vi "CRYChange Post Processing Data.vi"(8 "Step Setup VI No":i32, 9 "New Name":string[](array[string]), 10 "Old Name":string[](array[string]), 11 "Flatten Post Processing":string) -> (0 "Use Default Value":bool, 1 "Inserted Names Out":string[](array[string]), 2 "Original Names Out":string[](array[string]), 3 "Post Processing flattened Out":string)   [LabVIEW 2013]
uses:
  Typedef Control/CRYData Cluster Array.ctl
  Typedef Control/CRYData Cluster.ctl
  Typedef Control/CRYWaveform Cluster Array.ctl
  Typedef Control/CRYWaveform Cluster.ctl
  Typedef Control/CRYResult Cluster Array.ctl
  Typedef Control/CRYResult Cluster.ctl
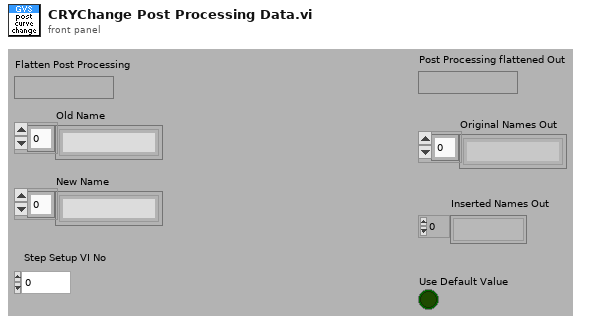
[diagram p1: front panel]
types:
  T1 = typedef "CRYPost Processing Cluster.ctl" = cluster{"Name":string, "Op Type":u16, "Curve A":string, "Curve B":string, "Axis Mode":u16, "Work Mode":u16, "Width":u16, "Weighting win":u16, "Search Mode":u16, "Freq Mode":u16, "New Sampling Rate":dbl, "Use Default Name":bool, "x":bool, "y":bool, "z":bool, "All points":bool, "A_single val axis":u16, "B_single val axis":u16, "Use Default Value":bool, "Result Name":string, "Smoothing Width":i32, "Window":u16, "Para_dB":sgl, "Para_%":sgl, "Exponent":sgl, "Hz":dbl, "Direct Weighting":bool, "Auto Inc":bool, "Inc(deg)":i32, "Total Rotation":i32, "Ref Freq Mode":u16, "Ref Waveform":string, "Sampling Rate":dbl, "Weighting Curve":string, "Ref Freq":dbl, "Curve Group":string[], "Search Items":string[], "Custom unit info":cluster{"use custom":bool, "lin/log":u16, "unit":string, "dB ref":dbl, "common dB":u16}, "Unit":string, "Type A":enum16{"Curves", "Values", "Results", "WFM"}, "Type B":enum16{"Curves", "Values", "Results", "WFM"}, "Unary Operator":u16, "Binary Operator":u16, "Statistical Operator":u16, "Constant ":dbl, "New Resolution":u16, "user equation cluster":T2, "Help":string, "Tab Value":enum32{"Setting", "Help"}, "Zwciker_X-axis":u16, "Zwicker_spectrum":bool, "Freq Sampling Mode":u16, "Freq Sampling Rate":dbl, "Smoothing":bool, "Work in Statics":u16, "Result Data":string[]}
  T2 = typedef "CRYUser Equation Cluster.ctl" = cluster{"Custom unit input array":cluster{"use custom":bool, "lin/log":u16, "unit":string, "dB ref":dbl, "common dB":u16}[], "Custom unit results array ":cluster{"use custom":bool, "lin/log":u16, "unit":string, "dB ref":dbl, "common dB":u16}[], "Desired Result Variables":string[], "Desired Result Names":string[], "Input Curve Names":string[], "Input Curve Variables":string[], "equation":string, "Input axis":u16[], "Results axis":u16[], "# input curves":i32, "# Desired result curves ":i32, "Input Values":string[], "Result Values":string[]}
  T3 = typedef "CRYResult Cluster Array.ctl" = T4[]
  T4 = typedef "CRYResult Cluster.ctl" = cluster{"Name":string, "Margin":dbl, "unit":string, "Verdict":bool, "Limit":string, "Max/Min":string, "protected":bool, "Step No.":i32, "Test Info":string, "AutoProtect":bool}
  T5 = typedef "CRYWaveform Cluster Array.ctl" = T6[]
  T6 = typedef "CRYWaveform Cluster.ctl" = cluster{"Waveform":cluster{"X0":dbl, "dX":dbl, "Y":sgl[]}, "X data":u16, "Y data":u16, "Y axis":u16, "X unit":string, "Y unit":string, "Y dB ref":dbl, "display Y":bool, "display X":bool, "Overload?":bool, "Test Info":string, "Step No.":i32, "Name":string, "protected":bool, "Sqc history":string[], "Signal Channel ID":i32, "Plot Settings":cluster{"Color":u32, "Interpolation":u8, "Point Style":u8, "Line Style":u8, "Point Color":u32, "Line Width":u8, "Bar Plot Style":u8, "Fill To":i16}, "AutoProtect":bool}
  T7 = typedef "CRYData Cluster Array.ctl" = T8[]
  T8 = typedef "CRYData Cluster.ctl" = cluster{"Name":string, "Curve":cluster{"x":dbl, "y":dbl, "z":dbl}[], "X data":u16, "Y data":u16, "Z data":u16, "X axis":u16, "Y axis":u16, "Z axis":u16, "X unit":string, "Y unit":string, "Z unit":string, "X dB ref":dbl, "Y dB ref":dbl, "Z dB ref":dbl, "single val":bool, "protected":bool, "display X":bool, "display Y":bool, "display Z":bool, "Test Info":string, "Step No.":i32, "Plot Settings":cluster{"Color":u32, "Interpolation":u8, "Point Style":u8, "Line Style":u8, "Point Color":u32, "Line Width":u8, "Bar Plot Style":u8, "Fill To":i16}, "AutoProtect":bool}
  T9 = cluster{"Res Name":string, "Type out":enum16{"Curves", "Values", "Results", "WFM"}}[]
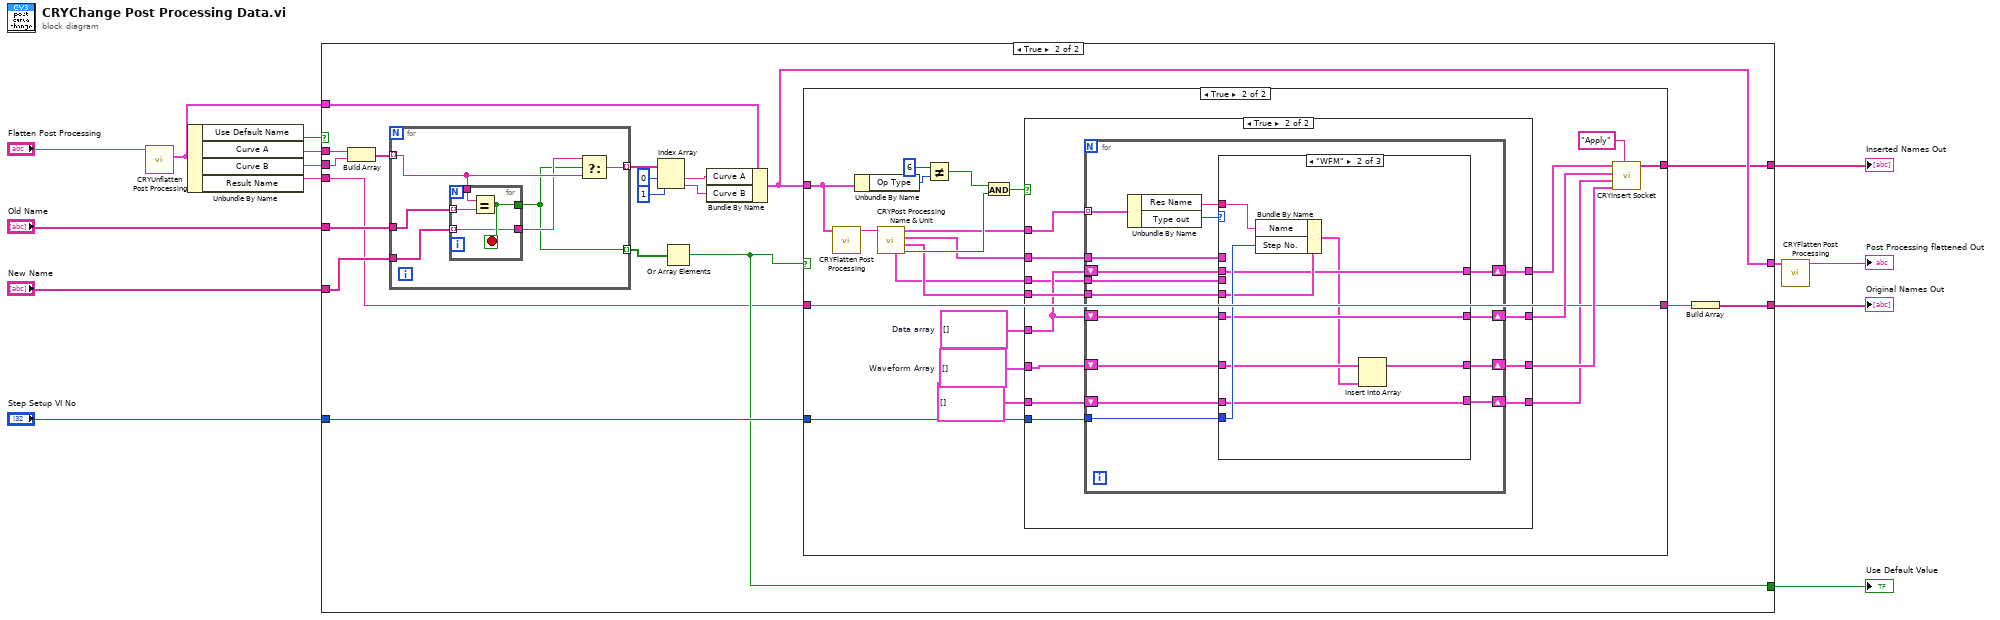
[diagram p0: block diagram]
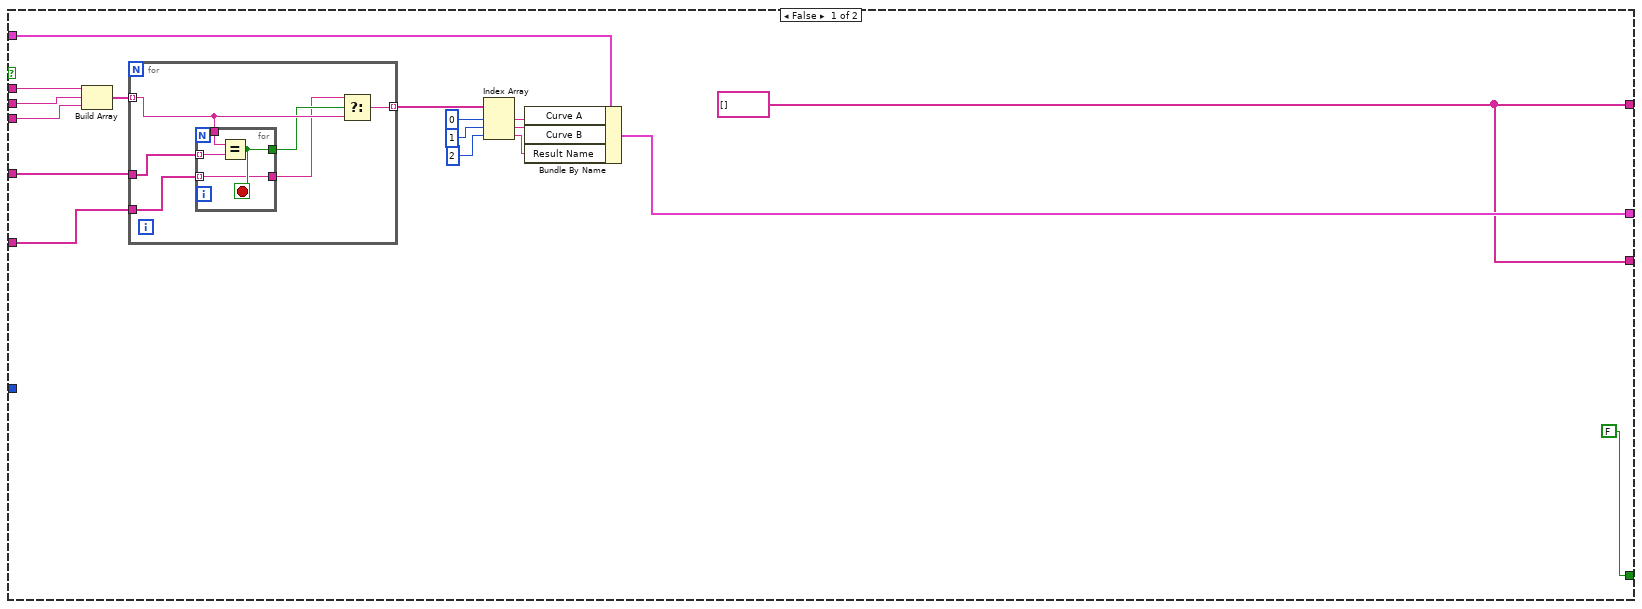
[diagram p2: hidden frame]
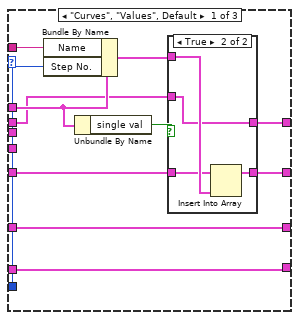
[diagram p5: hidden frame]
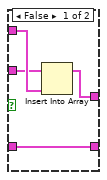
[diagram p6: hidden frame]
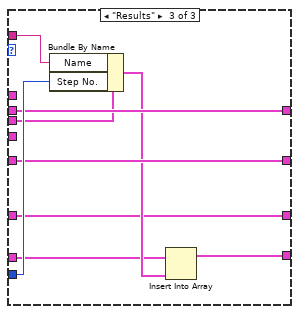
[diagram p7: hidden frame]
diagram:
  n1 = call "CRYUnflatten Post Processing.vi"("Unflatten Post Processing"="Flatten Post Processing") -> ("Post-Processing"=w8:T1)  [unwired: 8 in, 2 out]
  n2 = Unbundle By Name(w8) -> ("Use Default Name"=w9:bool, "Curve A"=w14:string, "Curve B"=w13:string, "Result Name"=w2:string)
  n3 = case shown="True" w9 {
    tunnel: w14 -> [w23 w60]
    tunnel: w13 -> [w22 w59]
    tunnel: [w17 w48] -> w12
    tunnel: w2 -> [w21 w44]
    tunnel: "Old Name" -> [w25 w52]
    tunnel: "New Name" -> [w24 w51]
    tunnel: w8 -> [w20 w50]
    tunnel: [w15 w47] -> w6
    tunnel: "Step Setup VI No" -> [_ w49]
    tunnel: [FALSE w45] -> w3
    tunnel: [w15 w42] -> w1
    frame False {
      w15 = string[] [] ("Inserted Names Out")
      n4 = Build Array(w23, w22, w21) -> (w31:string[])
      n5 = for {
        tunnel: w31 -> [w34] mode=indexing
        tunnel: w25 -> [w36]
        tunnel: [w37] -> w30 mode=indexing
        tunnel: w24 -> [w35]
        n6 = for {
          tunnel: w36 -> [w41] mode=indexing
          tunnel: [w39] -> w33
          tunnel: w34 -> [w40]
          tunnel: [w38] -> w32
          tunnel: w35 -> [w38] mode=indexing
          stop <- w39 stop-if-true
          n7 = Equal?(x=w40, y=w41) -> (x = y?=w39:bool)
        }
        n8 = Select(t=w32, s=w33, f=w34) -> (s? t:f=w37:string)
      }
      n9 = Index Array(array=w30, index #1=0 ("index"), index #2=1 ("index"), index #3=2 ("index")) -> (element #1=w27:string, element #2=w26:string, element #3=w18:string)
      n10 = Bundle By Name(cluster=w20, "Curve A"=w27, "Curve B"=w26, "Result Name"=w18) -> (w17:T1)
    }
    frame True {
      n11 = Build Array(w60, w59) -> (w58:string[])
      n12 = for {
        tunnel: w58 -> [w152] mode=indexing
        tunnel: w52 -> [w154]
        tunnel: [w155] -> w57 mode=indexing
        tunnel: w51 -> [w153]
        tunnel: [w150] -> w46 mode=indexing
        n13 = for {
          tunnel: w154 -> [w159] mode=indexing
          tunnel: [w157] -> w150
          tunnel: w152 -> [w158]
          tunnel: [w156] -> w151
          tunnel: w153 -> [w156] mode=indexing
          stop <- w157 stop-if-true
          n14 = Equal?(x=w158, y=w159) -> (x = y?=w157:bool)
        }
        n15 = Select(t=w151, s=w150, f=w152) -> (s? t:f=w155:string)
      }
      n16 = Index Array(array=w57, index #1=0 ("index"), index #2=1 ("index")) -> (element #1=w54:string, element #2=w53:string)
      n17 = Or Array Elements(Boolean array=w46) -> (logical OR=w45:bool)
      n18 = Bundle By Name(cluster=w50, "Curve A"=w54, "Curve B"=w53) -> (w48:T1)
      n19 = case shown="True" w45 {
        tunnel: w49 -> [_ w70]
        tunnel: w48 -> [_ w69]
        tunnel: [_ w65] -> w47
        tunnel: w44 -> [_ w64]
        tunnel: [_ w64] -> w43
        frame False {
        }
        frame True {
          w81 = T5 []  # Waveform Array
          w80 = T7 []  # Data array
          n20 = call "CRYFlatten Post Processing.vi"("Post-Processing"=w69) -> ("Post Processing flattened"=w71:string)  [unwired: 10 in]
          n21 = Unbundle By Name(w69) -> ("Op Type"=w72:u16)
          n22 = call "CRYPost Processing Name & Unit.vi"("Step setup"=w71) -> ("Run abble?"=w78:bool, "Waveform"=w76:T6, "Data"=w75:T8, "Result name and type"=w74:T9, "Result"=w62:T4)  [unwired: 6 in]
          n23 = Not Equal?(x=u16 6, y=w72) -> (x != y?=w77:bool)
          n24 = And(x=w77, y=w78) -> (x .and. y?=w79:bool)
          n25 = case shown="True" w79 {
            tunnel: w70 -> [_ w97]
            tunnel: [w85 w96] -> w68
            tunnel: [w85 w95] -> w67
            tunnel: [w84 w94] -> w66
            tunnel: w74 -> [_ w93]
            tunnel: w75 -> [_ w92]
            tunnel: w76 -> [_ w91]
            tunnel: w80 -> [w85 w90]
            tunnel: w81 -> [w84 w89]
            tunnel: T3 [] ("Results") -> [w83 w88]
            tunnel: w62 -> [_ w87]
            tunnel: [w83 w86] -> w61
            frame False {
            }
            frame True {
              n26 = for {
                tunnel: w93 -> [w112] mode=indexing
                tunnel: w97 -> [w110]
                tunnel: w91 -> [w109]
                tunnel: w92 -> [w108]
                shift-right: [w106] -> w94
                shift-left: w89 -> [w105]
                shift-right: [w103] -> w96
                shift-left: w90 -> [w104]
                shift-right: [w101] -> w95
                shift-left: w90 -> [w102]
                shift-right: [w98] -> w86
                shift-left: w88 -> [w100]
                tunnel: w87 -> [w99]
                n27 = Unbundle By Name(w112) -> ("Res Name"=w111:string, "Type out"=w107:enum16{"Curves", "Values", "Results", "WFM"})
                n28 = case shown="\"WFM\"" w107 {
                  tunnel: w111 -> [w123 w140 w149]
                  tunnel: w110 -> [w122 w139 w148]
                  tunnel: w109 -> [_ w138 _]
                  tunnel: w108 -> [w121 _ _]
                  tunnel: [w119 w136 w141] -> w106
                  tunnel: w105 -> [w119 w137 w141]
                  tunnel: w104 -> [w118 w135 w147]
                  tunnel: [w117 w135 w147] -> w103
                  tunnel: w102 -> [w116 w134 w146]
                  tunnel: [w115 w134 w146] -> w101
                  tunnel: w100 -> [w113 w132 w143]
                  tunnel: w99 -> [_ _ w144]
                  tunnel: [w113 w132 w142] -> w98
                  frame "Curves", "Values", Default {
                    n29 = Bundle By Name(cluster=w121, "Name"=w123, "Step No."=w122) -> (w114:T8)
                    n30 = Unbundle By Name(w121) -> ("single val"=w120:bool)
                    n31 = case shown="True" w120 {
                      tunnel: w114 -> [w127 w131]
                      tunnel: w118 -> [w126 w128]
                      tunnel: [w125 w128] -> w117
                      tunnel: w116 -> [w124 w130]
                      tunnel: [w124 w129] -> w115
                      frame False {
                        n32 = Insert Into Array(array=w126, new element=w127) -> (w125:T7)  [unwired: 1 in]
                      }
                      frame True {
                        n33 = Insert Into Array(array=w130, new element=w131) -> (w129:T7)  [unwired: 1 in]
                      }
                    }
                  }
                  frame "WFM" {
                    n34 = Bundle By Name(cluster=w138, "Name"=w140, "Step No."=w139) -> (w133:T6)
                    n35 = Insert Into Array(array=w137, new element=w133) -> (w136:T5)  [unwired: 1 in]
                  }
                  frame "Results" {
                    n36 = Bundle By Name(cluster=w144, "Name"=w149, "Step No."=w148) -> (w145:T4)
                    n37 = Insert Into Array(array=w143, new element=w145) -> (w142:T3)  [unwired: 1 in]
                  }
                }
              }
            }
          }
          n38 = call "CRYInsert Socket.vi"("sOption1"="Apply", "Waves"=w66, "Results"=w61, "Values"=w67, "Curves"=w68) -> ("Inserted Names Out"=w65:string[])  [unwired: 6 in]
        }
      }
      n39 = Build Array(w43) -> (w42:string[])
    }
  }
  "Inserted Names Out" <- w6
  "Use Default Value" <- w3
  "Original Names Out" <- w1
  n40 = call "CRYFlatten Post Processing.vi"("Post-Processing"=w12) -> ("Post Processing flattened"=→"Post Processing flattened Out":string)  [unwired: 10 in]
